vi "Untitled 1.vi"() -> ()   [LabVIEW 2019]
panel:
  out "Load Successful?":bool
  out "size(s)":i32
  in  "OK Button 2":bool
  out "element":string
  in  "Load new stations":bool
  in  "Line name":string
  in  "Line stations":string[](array[string])
  out "read buffer":string
  in  "VISA resource name":refnum<visa-resource-name>
  in  "Stop program":bool
  out "End\nStation":bool caption="N/A"
  out "Station 15":bool caption="N/A"
  out "Station 14":bool caption="N/A"
  out "Station 13":bool caption="N/A"
  out "Station 12":bool caption="N/A"
  out "Station 11":bool caption="N/A"
  out "Station 10":bool caption="N/A"
  out "Station 9":bool caption="N/A"
  out "Station 8":bool caption="N/A"
  out "Station 7":bool caption="sevsv"
  out "Station 6":bool caption="iugg"
  out "Station 5":bool caption="esceac"
  out "Station 4":bool caption="dwafa"
  out "Station 3":bool caption="wdca"
  out "Station 2":bool caption="kugiyg"
  out "Starting\nStation":bool caption="khfydug"
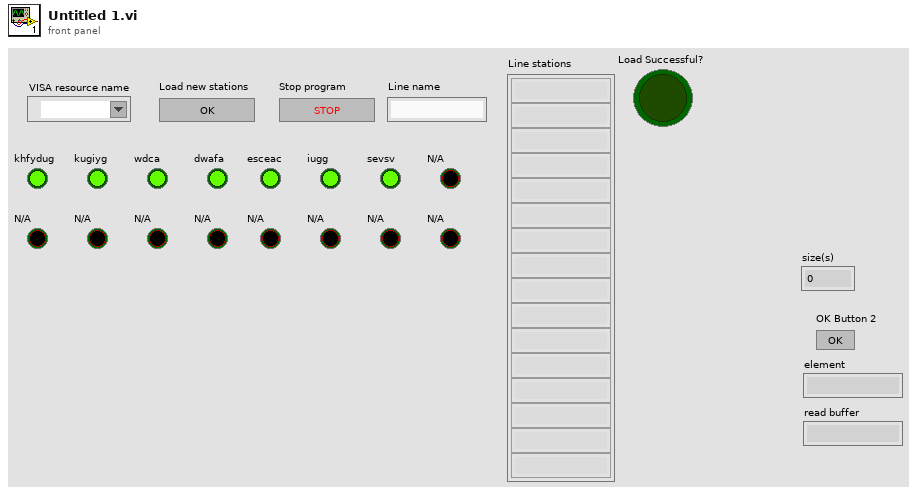
[diagram p1: front panel]
types:
  T1 = enum8{"Enabled", "Disabled", "Disabled and Grayed Out"}
  T2 = cluster{"[0]":bool, "[1]":bool, "[2]":bool, "[3]":bool, "[4]":bool, "[5]":bool, "[6]":bool, "[7]":bool, "[8]":bool}
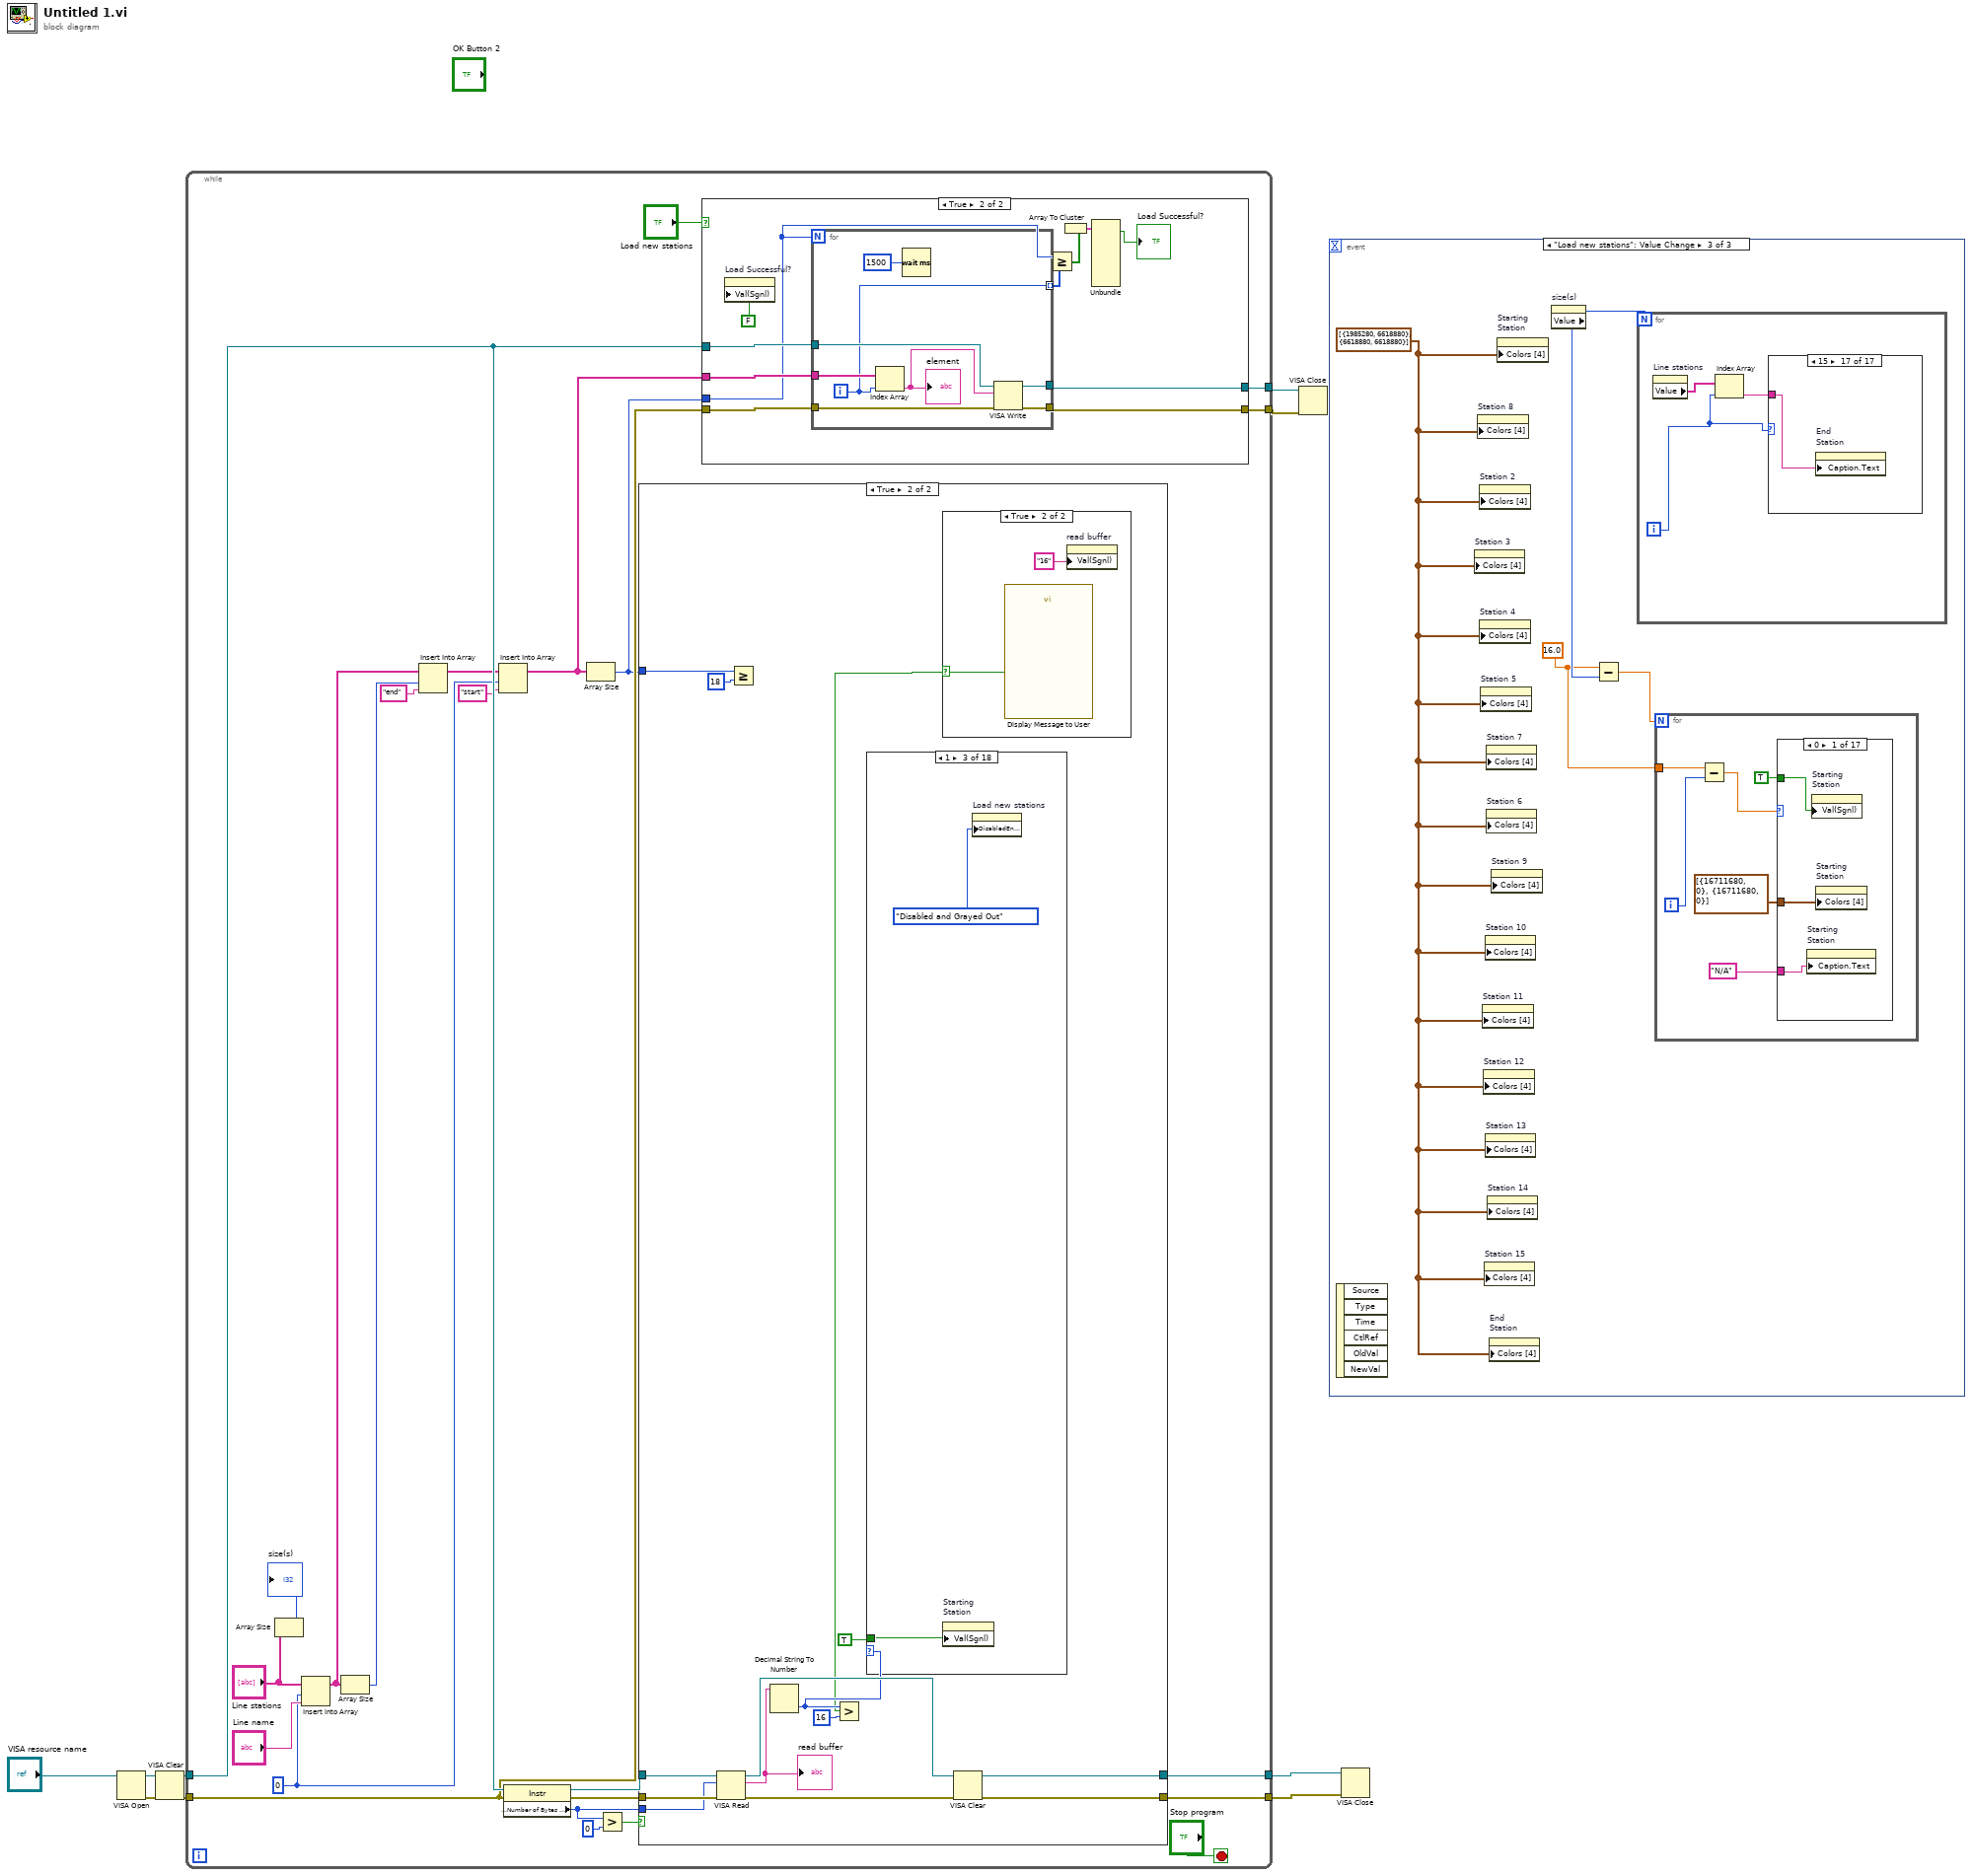
[diagram p0: block diagram]
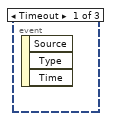
[diagram p2: hidden frame]
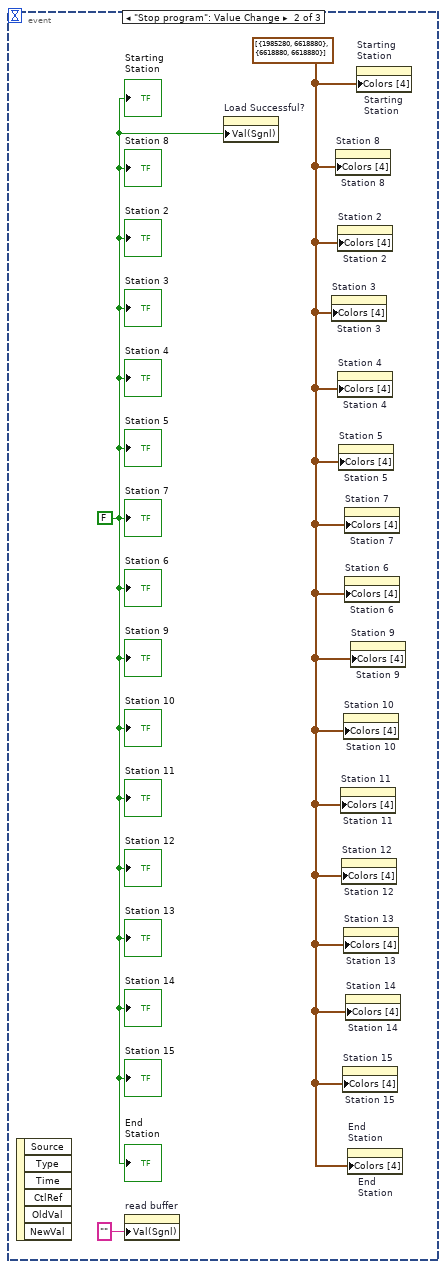
[diagram p3: hidden frame]
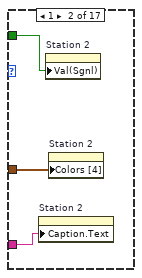
[diagram p4: hidden frame]
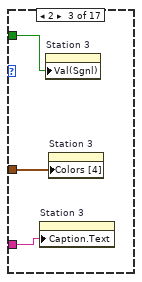
[diagram p5: hidden frame]
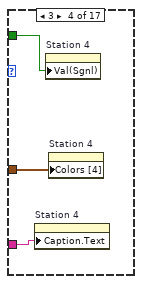
[diagram p6: hidden frame]
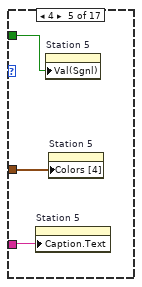
[diagram p7: hidden frame]
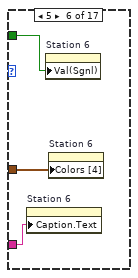
[diagram p8: hidden frame]
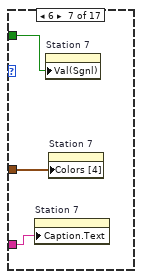
[diagram p9: hidden frame]
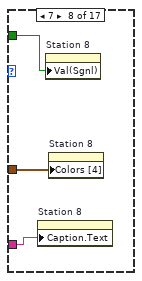
[diagram p10: hidden frame]
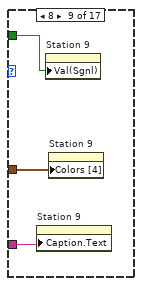
[diagram p11: hidden frame]
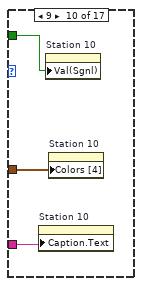
[diagram p12: hidden frame]
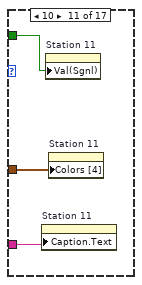
[diagram p13: hidden frame]
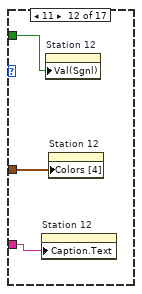
[diagram p14: hidden frame]
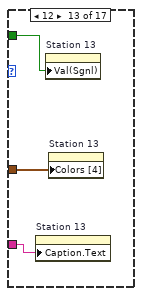
[diagram p15: hidden frame]
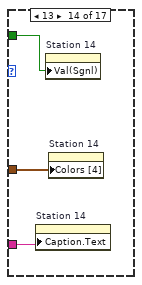
[diagram p16: hidden frame]
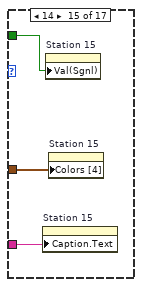
[diagram p17: hidden frame]
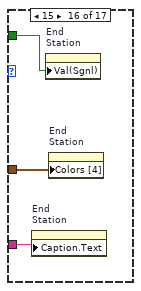
[diagram p18: hidden frame]
diagram:
  n1 = VISA Open(VISA resource name="VISA resource name") -> (VISA resource name=w5:refnum<visa-resource-name>, error out=w6:errorcluster)  [unwired: 4 in]
  n2 = VISA Clear(VISA resource name=w5, error in (no error)=w6) -> (VISA resource name out=w4:refnum<visa-resource-name>, error out=w3:errorcluster)
  n3 = while {
    tunnel: w4 -> [w21]
    tunnel: w3 -> [w20]
    tunnel: [w28] -> w8
    tunnel: [w27] -> w7
    tunnel: [w16] -> w2
    tunnel: [w15] -> w1
    stop <- "Stop program" stop-if-true
    w14 = 0 ("index")
    n4 = Array Size(array="Line stations") -> (size(s)=→"size(s)":i32)
    n5 = Insert Into Array(array="Line stations", index=w14, new element="Line name") -> (w22:string[])
    n6 = Array Size(array=w22) -> (size(s)=w23:i32)
    n7 = Insert Into Array(array=w22, index=w23, new element="end") -> (w18:string[])
    n8 = Insert Into Array(array=w18, index=w14, new element="start" ("new element/subarray")) -> (w13:string[])
    n9 = property class="Instr"(reference=w21, error in=w20) -> (reference out=w31:refnum<visa-resource-name>, error out=w30:errorcluster, "Serial Settings:Number of Bytes at Serial Port"=w29:u32)
    n10 = Array Size(array=w13) -> (size(s)=w12:i32)
    n11 = Greater?(x=w29, y=u32 0) -> (0:w32:bool)
    n12 = case shown="True" w32 {
      tunnel: w31 -> [w56 w70]
      tunnel: w30 -> [w55 w69]
      tunnel: [w56 w67] -> w27
      tunnel: [w55 w64] -> w28
      tunnel: w29 -> [_ w68]
      tunnel: w12 -> [_ w59]
      frame False {
      }
      frame True {
        n13 = VISA Read(VISA resource name=w70, byte count=w68, error in (no error)=w69) -> (VISA resource name out=w66:refnum<visa-resource-name>, read buffer=w63:string, error out=w65:errorcluster)  [unwired: 1 out]
        "read buffer" <- w63
        n14 = Greater Or Equal?(x=w59, y=18) -> ()  [unwired: 1 out]
        n15 = Decimal String To Number(string=w63) -> (number=w60:i32)  [unwired: 2 in, 1 out]
        n16 = Greater?(x=w60, y=16) -> (0:w57:bool)
        n17 = case shown="1" w60 {
          tunnel: TRUE -> [_ _ w76 w77 w78 w79 w80 w81 w82 w83 w84 w85 w86 w87 w88 w89 w90 w91]
          frame Default {
          }
          frame 0 {
            w73 = FALSE
            n18 = property on="Load new stations" class="Bool"("DisabledEnum"=T1."Enabled" ("Disabled")) -> ()  [unwired: 2 in, 2 out]
            n19 = property on="Station 5" class="Bool (strict)"("Val(Sgnl)"=w73) -> ()  [unwired: 2 in, 2 out]
            n20 = property on="Station 4" class="Bool (strict)"("Val(Sgnl)"=w73) -> ()  [unwired: 2 in, 2 out]
            n21 = property on="Station 6" class="Bool (strict)"("Val(Sgnl)"=w73) -> ()  [unwired: 2 in, 2 out]
            n22 = property on="Station 3" class="Bool (strict)"("Val(Sgnl)"=w73) -> ()  [unwired: 2 in, 2 out]
            n23 = property on="Starting\nStation" class="Bool (strict)"("Val(Sgnl)"=w73) -> ()  [unwired: 2 in, 2 out]
            n24 = property on="Station 2" class="Bool (strict)"("Val(Sgnl)"=w73) -> ()  [unwired: 2 in, 2 out]
            n25 = property on="Station 7" class="Bool (strict)"("Val(Sgnl)"=w73) -> ()  [unwired: 2 in, 2 out]
            n26 = property on="Station 11" class="Bool (strict)"("Val(Sgnl)"=w73) -> ()  [unwired: 2 in, 2 out]
            n27 = property on="Station 12" class="Bool (strict)"("Val(Sgnl)"=w73) -> ()  [unwired: 2 in, 2 out]
            n28 = property on="Station 10" class="Bool (strict)"("Val(Sgnl)"=w73) -> ()  [unwired: 2 in, 2 out]
            n29 = property on="Station 9" class="Bool (strict)"("Val(Sgnl)"=w73) -> ()  [unwired: 2 in, 2 out]
            n30 = property on="Station 8" class="Bool (strict)"("Val(Sgnl)"=w73) -> ()  [unwired: 2 in, 2 out]
            n31 = property on="Station 15" class="Bool (strict)"("Val(Sgnl)"=w73) -> ()  [unwired: 2 in, 2 out]
            n32 = property on="Station 13" class="Bool (strict)"("Val(Sgnl)"=w73) -> ()  [unwired: 2 in, 2 out]
            n33 = property on="End\nStation" class="Bool (strict)"("Val(Sgnl)"=w73) -> ()  [unwired: 2 in, 2 out]
            n34 = property on="Station 14" class="Bool (strict)"("Val(Sgnl)"=w73) -> ()  [unwired: 2 in, 2 out]
          }
          frame 1 {
            n35 = property on="Starting\nStation" class="Bool (strict)"("Val(Sgnl)"=w76) -> ()  [unwired: 2 in, 2 out]
            n36 = property on="Load new stations" class="Bool"("DisabledEnum"=T1."Disabled and Grayed Out" ("Disabled")) -> ()  [unwired: 2 in, 2 out]
          }
          frame 2 {
            n37 = property on="Station 2" class="Bool (strict)"("Val(Sgnl)"=w77) -> ()  [unwired: 2 in, 2 out]
          }
          frame 3 {
            n38 = property on="Station 3" class="Bool (strict)"("Val(Sgnl)"=w78) -> ()  [unwired: 2 in, 2 out]
          }
          frame 4 {
            n39 = property on="Station 4" class="Bool (strict)"("Val(Sgnl)"=w79) -> ()  [unwired: 2 in, 2 out]
          }
          frame 5 {
            n40 = property on="Station 5" class="Bool (strict)"("Val(Sgnl)"=w80) -> ()  [unwired: 2 in, 2 out]
          }
          frame 6 {
            n41 = property on="Station 6" class="Bool (strict)"("Val(Sgnl)"=w81) -> ()  [unwired: 2 in, 2 out]
          }
          frame 7 {
            n42 = property on="Station 7" class="Bool (strict)"("Val(Sgnl)"=w82) -> ()  [unwired: 2 in, 2 out]
          }
          frame 8 {
            n43 = property on="Station 8" class="Bool (strict)"("Val(Sgnl)"=w83) -> ()  [unwired: 2 in, 2 out]
          }
          frame 9 {
            n44 = property on="Station 9" class="Bool (strict)"("Val(Sgnl)"=w84) -> ()  [unwired: 2 in, 2 out]
          }
          frame 10 {
            n45 = property on="Station 10" class="Bool (strict)"("Val(Sgnl)"=w85) -> ()  [unwired: 2 in, 2 out]
          }
          frame 11 {
            n46 = property on="Station 11" class="Bool (strict)"("Val(Sgnl)"=w86) -> ()  [unwired: 2 in, 2 out]
          }
          frame 12 {
            n47 = property on="Station 12" class="Bool (strict)"("Val(Sgnl)"=w87) -> ()  [unwired: 2 in, 2 out]
          }
          frame 13 {
            n48 = property on="Station 13" class="Bool (strict)"("Val(Sgnl)"=w88) -> ()  [unwired: 2 in, 2 out]
          }
          frame 14 {
            n49 = property on="Station 14" class="Bool (strict)"("Val(Sgnl)"=w89) -> ()  [unwired: 2 in, 2 out]
          }
          frame 15 {
            n50 = property on="Station 15" class="Bool (strict)"("Val(Sgnl)"=w90) -> ()  [unwired: 2 in, 2 out]
          }
          frame 16 {
            n51 = property on="End\nStation" class="Bool (strict)"("Val(Sgnl)"=w91) -> ()  [unwired: 2 in, 2 out]
          }
        }
        n52 = case shown="True" w57 {
          selector: w57 -> [_ w72]
          frame False {
          }
          frame True {
            n53 = call "Display Message to User"("Enable"=w72) -> ()  [unwired: 9 in, 2 out]
            n54 = property on="read buffer" class="Str"("Val(Sgnl)"="16" ("Value (Signaling)")) -> ()  [unwired: 2 in, 2 out]
          }
        }
        n55 = VISA Clear(VISA resource name=w66, error in (no error)=w65) -> (VISA resource name out=w67:refnum<visa-resource-name>, error out=w64:errorcluster)
      }
    }
    n56 = case shown="True" "Load new stations" {
      tunnel: w21 -> [w35 w45]
      tunnel: w20 -> [w34 w44]
      tunnel: w13 -> [_ w46]
      tunnel: [w35 w43] -> w16
      tunnel: [w34 w42] -> w15
      tunnel: w12 -> [_ w41]
      frame False {
      }
      frame True {
        n57 = property on="Load Successful?" class="Bool (strict)"("Val(Sgnl)"=FALSE ("Value (Signaling)")) -> ()  [unwired: 2 in, 2 out]
        n58 = for {
          N: w41 -> [_]
          tunnel: w46 -> [w54]
          tunnel: w45 -> [w53]
          tunnel: w44 -> [w52]
          tunnel: [w50] -> w43
          tunnel: [w49] -> w42
          tunnel: [w47] -> w40 mode=indexing
          i -> [w47]
          n59 = Index Array(array=w54, index=w47) -> (element=w51:string)
          "element" <- w51
          n60 = Wait (ms)(milliseconds to wait=u32 1500) -> ()  [unwired: 1 out]
          n61 = VISA Write(VISA resource name=w53, write buffer=w51, error in (no error)=w52) -> (VISA resource name out=w50:refnum<visa-resource-name>, error out=w49:errorcluster)  [unwired: 1 out]
        }
        n62 = Greater Or Equal?(x=w41, y=w40) -> (x >= y?=w39:bool[])
        n63 = Array To Cluster(array=w39) -> (cluster=w38:T2)
        n64 = Unbundle(w38) -> ("[1]"=→"Load Successful?":bool)  [unwired: 8 out]
      }
    }
  }
  n65 = VISA Close(VISA resource name=w2, error in (no error)=w1) -> ()  [unwired: 1 out]
  n66 = event shown="[2] \"Load new stations\": Value Change" {
    selector: _ -> [_ _ _]
    dyn-events: _ -> [_ _ _]
    timeout: _ -> [_ _ _]
    event Timeout {
      n67 = event-data() -> ()  [unwired: 1 in, 3 out]
    }
    event "Stop program": Value Change {
      w93 = cluster{u32, u32}[] [{1985280, 6618880}, {6618880, 6618880}] ("Colors [4]")
      w94 = cluster{u32, u32}[] [{1985280, 6618880}, {6618880, 6618880}] ("Colors [4]")
      w92 = FALSE
      n68 = event-data() -> ()  [unwired: 1 in, 6 out]
      n69 = property on="read buffer" class="Str"("Val(Sgnl)"="" ("Value (Signaling)")) -> ()  [unwired: 2 in, 2 out]
      n70 = property on="Load Successful?" class="Bool (strict)"("Val(Sgnl)"=w92) -> ()  [unwired: 2 in, 2 out]
      n71 = property on="Station 3" class="Bool (strict)"("Colors [4]"=w93) -> ()  [unwired: 2 in, 2 out]
      n72 = property on="Station 3" class="Bool (strict)"("Colors [4]"=w94) -> ()  [unwired: 2 in, 2 out]
      n73 = property on="Station 8" class="Bool (strict)"("Colors [4]"=w93) -> ()  [unwired: 2 in, 2 out]
      n74 = property on="Station 8" class="Bool (strict)"("Colors [4]"=w94) -> ()  [unwired: 2 in, 2 out]
      n75 = property on="Station 2" class="Bool (strict)"("Colors [4]"=w93) -> ()  [unwired: 2 in, 2 out]
      n76 = property on="Station 2" class="Bool (strict)"("Colors [4]"=w94) -> ()  [unwired: 2 in, 2 out]
      n77 = property on="Station 4" class="Bool (strict)"("Colors [4]"=w93) -> ()  [unwired: 2 in, 2 out]
      n78 = property on="Station 4" class="Bool (strict)"("Colors [4]"=w94) -> ()  [unwired: 2 in, 2 out]
      n79 = property on="Station 5" class="Bool (strict)"("Colors [4]"=w93) -> ()  [unwired: 2 in, 2 out]
      n80 = property on="Station 5" class="Bool (strict)"("Colors [4]"=w94) -> ()  [unwired: 2 in, 2 out]
      n81 = property on="Station 11" class="Bool (strict)"("Colors [4]"=w93) -> ()  [unwired: 2 in, 2 out]
      n82 = property on="Station 11" class="Bool (strict)"("Colors [4]"=w94) -> ()  [unwired: 2 in, 2 out]
      n83 = property on="Station 12" class="Bool (strict)"("Colors [4]"=w93) -> ()  [unwired: 2 in, 2 out]
      n84 = property on="Station 12" class="Bool (strict)"("Colors [4]"=w94) -> ()  [unwired: 2 in, 2 out]
      n85 = property on="Station 15" class="Bool (strict)"("Colors [4]"=w93) -> ()  [unwired: 2 in, 2 out]
      n86 = property on="Station 15" class="Bool (strict)"("Colors [4]"=w94) -> ()  [unwired: 2 in, 2 out]
      n87 = property on="Station 10" class="Bool (strict)"("Colors [4]"=w93) -> ()  [unwired: 2 in, 2 out]
      n88 = property on="Station 10" class="Bool (strict)"("Colors [4]"=w94) -> ()  [unwired: 2 in, 2 out]
      n89 = property on="Station 13" class="Bool (strict)"("Colors [4]"=w93) -> ()  [unwired: 2 in, 2 out]
      n90 = property on="Station 13" class="Bool (strict)"("Colors [4]"=w94) -> ()  [unwired: 2 in, 2 out]
      n91 = property on="Station 7" class="Bool (strict)"("Colors [4]"=w93) -> ()  [unwired: 2 in, 2 out]
      n92 = property on="Station 7" class="Bool (strict)"("Colors [4]"=w94) -> ()  [unwired: 2 in, 2 out]
      n93 = property on="Station 6" class="Bool (strict)"("Colors [4]"=w93) -> ()  [unwired: 2 in, 2 out]
      n94 = property on="Station 6" class="Bool (strict)"("Colors [4]"=w94) -> ()  [unwired: 2 in, 2 out]
      n95 = property on="Station 14" class="Bool (strict)"("Colors [4]"=w93) -> ()  [unwired: 2 in, 2 out]
      n96 = property on="Station 14" class="Bool (strict)"("Colors [4]"=w94) -> ()  [unwired: 2 in, 2 out]
      n97 = property on="End\nStation" class="Bool (strict)"("Colors [4]"=w93) -> ()  [unwired: 2 in, 2 out]
      n98 = property on="End\nStation" class="Bool (strict)"("Colors [4]"=w94) -> ()  [unwired: 2 in, 2 out]
      n99 = property on="Station 9" class="Bool (strict)"("Colors [4]"=w93) -> ()  [unwired: 2 in, 2 out]
      n100 = property on="Station 9" class="Bool (strict)"("Colors [4]"=w94) -> ()  [unwired: 2 in, 2 out]
      n101 = property on="Starting\nStation" class="Bool (strict)"("Colors [4]"=w93) -> ()  [unwired: 2 in, 2 out]
      n102 = property on="Starting\nStation" class="Bool (strict)"("Colors [4]"=w94) -> ()  [unwired: 2 in, 2 out]
      "Station 2" <- w92
      "Station 3" <- w92
      "Station 4" <- w92
      "Station 5" <- w92
      "Station 6" <- w92
      "Station 7" <- w92
      "Station 8" <- w92
      "Station 9" <- w92
      "Station 10" <- w92
      "Station 11" <- w92
      "Station 12" <- w92
      "Station 13" <- w92
      "Station 14" <- w92
      "Station 15" <- w92
      "End\nStation" <- w92
      "Starting\nStation" <- w92
    }
    event "Load new stations": Value Change {
      w96 = cluster{u32, u32}[] [{1985280, 6618880}, {6618880, 6618880}] ("Colors [4]")
      w97 = 16.0 ("x")
      n103 = event-data() -> ()  [unwired: 1 in, 6 out]
      n104 = property on="Station 3" class="Bool (strict)"("Colors [4]"=w96) -> ()  [unwired: 2 in, 2 out]
      n105 = property on="Station 8" class="Bool (strict)"("Colors [4]"=w96) -> ()  [unwired: 2 in, 2 out]
      n106 = property on="Station 2" class="Bool (strict)"("Colors [4]"=w96) -> ()  [unwired: 2 in, 2 out]
      n107 = property on="Station 4" class="Bool (strict)"("Colors [4]"=w96) -> ()  [unwired: 2 in, 2 out]
      n108 = property on="Station 5" class="Bool (strict)"("Colors [4]"=w96) -> ()  [unwired: 2 in, 2 out]
      n109 = property on="Station 11" class="Bool (strict)"("Colors [4]"=w96) -> ()  [unwired: 2 in, 2 out]
      n110 = property on="Station 12" class="Bool (strict)"("Colors [4]"=w96) -> ()  [unwired: 2 in, 2 out]
      n111 = property on="Station 15" class="Bool (strict)"("Colors [4]"=w96) -> ()  [unwired: 2 in, 2 out]
      n112 = property on="Station 10" class="Bool (strict)"("Colors [4]"=w96) -> ()  [unwired: 2 in, 2 out]
      n113 = property on="Station 13" class="Bool (strict)"("Colors [4]"=w96) -> ()  [unwired: 2 in, 2 out]
      n114 = property on="Station 7" class="Bool (strict)"("Colors [4]"=w96) -> ()  [unwired: 2 in, 2 out]
      n115 = property on="Station 6" class="Bool (strict)"("Colors [4]"=w96) -> ()  [unwired: 2 in, 2 out]
      n116 = property on="Station 14" class="Bool (strict)"("Colors [4]"=w96) -> ()  [unwired: 2 in, 2 out]
      n117 = property on="End\nStation" class="Bool (strict)"("Colors [4]"=w96) -> ()  [unwired: 2 in, 2 out]
      n118 = property on="Station 9" class="Bool (strict)"("Colors [4]"=w96) -> ()  [unwired: 2 in, 2 out]
      n119 = property on="Starting\nStation" class="Bool (strict)"("Colors [4]"=w96) -> ()  [unwired: 2 in, 2 out]
      n120 = property on="size(s)" class="DigNum (strict)"() -> ("Value"=w99:i32)  [unwired: 2 in, 2 out]
      n121 = Subtract(x=w97, y=w99) -> (x-y=w98:dbl)
      n122 = for {
        N: w99 -> [_]
        i -> [w154]
        n123 = property on="Line stations" class="Arr (strict)"() -> ("Value"=w156:string[])  [unwired: 2 in, 2 out]
        n124 = Index Array(array=w156, index=w154) -> (element=w155:string)
        n125 = case shown="15" w154 {
          tunnel: w155 -> [_ w157 w158 w159 w160 w161 w162 w163 w164 w165 w166 w167 w168 w169 w170 w171 w172]
          frame Default {
          }
          frame 0 {
            n126 = property on="Starting\nStation" class="Bool (strict)"("Caption.Text"=w157) -> ()  [unwired: 2 in, 2 out]
          }
          frame 1 {
            n127 = property on="Station 2" class="Bool (strict)"("Caption.Text"=w158) -> ()  [unwired: 2 in, 2 out]
          }
          frame 2 {
            n128 = property on="Station 3" class="Bool (strict)"("Caption.Text"=w159) -> ()  [unwired: 2 in, 2 out]
          }
          frame 3 {
            n129 = property on="Station 4" class="Bool (strict)"("Caption.Text"=w160) -> ()  [unwired: 2 in, 2 out]
          }
          frame 4 {
            n130 = property on="Station 5" class="Bool (strict)"("Caption.Text"=w161) -> ()  [unwired: 2 in, 2 out]
          }
          frame 5 {
            n131 = property on="Station 6" class="Bool (strict)"("Caption.Text"=w162) -> ()  [unwired: 2 in, 2 out]
          }
          frame 6 {
            n132 = property on="Station 7" class="Bool (strict)"("Caption.Text"=w163) -> ()  [unwired: 2 in, 2 out]
          }
          frame 7 {
            n133 = property on="Station 8" class="Bool (strict)"("Caption.Text"=w164) -> ()  [unwired: 2 in, 2 out]
          }
          frame 8 {
            n134 = property on="Station 9" class="Bool (strict)"("Caption.Text"=w165) -> ()  [unwired: 2 in, 2 out]
          }
          frame 9 {
            n135 = property on="Station 10" class="Bool (strict)"("Caption.Text"=w166) -> ()  [unwired: 2 in, 2 out]
          }
          frame 10 {
            n136 = property on="Station 11" class="Bool (strict)"("Caption.Text"=w167) -> ()  [unwired: 2 in, 2 out]
          }
          frame 11 {
            n137 = property on="Station 12" class="Bool (strict)"("Caption.Text"=w168) -> ()  [unwired: 2 in, 2 out]
          }
          frame 12 {
            n138 = property on="Station 13" class="Bool (strict)"("Caption.Text"=w169) -> ()  [unwired: 2 in, 2 out]
          }
          frame 13 {
            n139 = property on="Station 14" class="Bool (strict)"("Caption.Text"=w170) -> ()  [unwired: 2 in, 2 out]
          }
          frame 14 {
            n140 = property on="Station 15" class="Bool (strict)"("Caption.Text"=w171) -> ()  [unwired: 2 in, 2 out]
          }
          frame 15 {
            n141 = property on="End\nStation" class="Bool (strict)"("Caption.Text"=w172) -> ()  [unwired: 2 in, 2 out]
          }
        }
      }
      n142 = for {
        N: w98 -> [_]
        tunnel: w97 -> [w105]
        i -> [w104]
        n143 = Subtract(x=w105, y=w104) -> (x-y=w103:dbl)
        n144 = case shown="0" w103 {
          tunnel: cluster{u32, u32}[] [{16711680, 0}, {16711680, 0}] ("Colors [4]") -> [w108 w111 w114 w117 w120 w123 w126 w129 w132 w135 w138 w141 w144 w147 w150 w153 _]
          tunnel: TRUE ("Value (Signaling)") -> [w107 w110 w113 w116 w119 w122 w125 w128 w131 w134 w137 w140 w143 w146 w149 w152 _]
          tunnel: "N/A" ("Caption.Text") -> [w106 w109 w112 w115 w118 w121 w124 w127 w130 w133 w136 w139 w142 w145 w148 w151 _]
          frame 0 {
            n145 = property on="Starting\nStation" class="Bool (strict)"("Caption.Text"=w106) -> ()  [unwired: 2 in, 2 out]
            n146 = property on="Starting\nStation" class="Bool (strict)"("Val(Sgnl)"=w107) -> ()  [unwired: 2 in, 2 out]
            n147 = property on="Starting\nStation" class="Bool (strict)"("Colors [4]"=w108) -> ()  [unwired: 2 in, 2 out]
          }
          frame 1 {
            n148 = property on="Station 2" class="Bool (strict)"("Caption.Text"=w109) -> ()  [unwired: 2 in, 2 out]
            n149 = property on="Station 2" class="Bool (strict)"("Val(Sgnl)"=w110) -> ()  [unwired: 2 in, 2 out]
            n150 = property on="Station 2" class="Bool (strict)"("Colors [4]"=w111) -> ()  [unwired: 2 in, 2 out]
          }
          frame 2 {
            n151 = property on="Station 3" class="Bool (strict)"("Caption.Text"=w112) -> ()  [unwired: 2 in, 2 out]
            n152 = property on="Station 3" class="Bool (strict)"("Val(Sgnl)"=w113) -> ()  [unwired: 2 in, 2 out]
            n153 = property on="Station 3" class="Bool (strict)"("Colors [4]"=w114) -> ()  [unwired: 2 in, 2 out]
          }
          frame 3 {
            n154 = property on="Station 4" class="Bool (strict)"("Caption.Text"=w115) -> ()  [unwired: 2 in, 2 out]
            n155 = property on="Station 4" class="Bool (strict)"("Val(Sgnl)"=w116) -> ()  [unwired: 2 in, 2 out]
            n156 = property on="Station 4" class="Bool (strict)"("Colors [4]"=w117) -> ()  [unwired: 2 in, 2 out]
          }
          frame 4 {
            n157 = property on="Station 5" class="Bool (strict)"("Caption.Text"=w118) -> ()  [unwired: 2 in, 2 out]
            n158 = property on="Station 5" class="Bool (strict)"("Val(Sgnl)"=w119) -> ()  [unwired: 2 in, 2 out]
            n159 = property on="Station 5" class="Bool (strict)"("Colors [4]"=w120) -> ()  [unwired: 2 in, 2 out]
          }
          frame 5 {
            n160 = property on="Station 6" class="Bool (strict)"("Caption.Text"=w121) -> ()  [unwired: 2 in, 2 out]
            n161 = property on="Station 6" class="Bool (strict)"("Val(Sgnl)"=w122) -> ()  [unwired: 2 in, 2 out]
            n162 = property on="Station 6" class="Bool (strict)"("Colors [4]"=w123) -> ()  [unwired: 2 in, 2 out]
          }
          frame 6 {
            n163 = property on="Station 7" class="Bool (strict)"("Caption.Text"=w124) -> ()  [unwired: 2 in, 2 out]
            n164 = property on="Station 7" class="Bool (strict)"("Val(Sgnl)"=w125) -> ()  [unwired: 2 in, 2 out]
            n165 = property on="Station 7" class="Bool (strict)"("Colors [4]"=w126) -> ()  [unwired: 2 in, 2 out]
          }
          frame 7 {
            n166 = property on="Station 8" class="Bool (strict)"("Caption.Text"=w127) -> ()  [unwired: 2 in, 2 out]
            n167 = property on="Station 8" class="Bool (strict)"("Val(Sgnl)"=w128) -> ()  [unwired: 2 in, 2 out]
            n168 = property on="Station 8" class="Bool (strict)"("Colors [4]"=w129) -> ()  [unwired: 2 in, 2 out]
          }
          frame 8 {
            n169 = property on="Station 9" class="Bool (strict)"("Caption.Text"=w130) -> ()  [unwired: 2 in, 2 out]
            n170 = property on="Station 9" class="Bool (strict)"("Val(Sgnl)"=w131) -> ()  [unwired: 2 in, 2 out]
            n171 = property on="Station 9" class="Bool (strict)"("Colors [4]"=w132) -> ()  [unwired: 2 in, 2 out]
          }
          frame 9 {
            n172 = property on="Station 10" class="Bool (strict)"("Caption.Text"=w133) -> ()  [unwired: 2 in, 2 out]
            n173 = property on="Station 10" class="Bool (strict)"("Val(Sgnl)"=w134) -> ()  [unwired: 2 in, 2 out]
            n174 = property on="Station 10" class="Bool (strict)"("Colors [4]"=w135) -> ()  [unwired: 2 in, 2 out]
          }
          frame 10 {
            n175 = property on="Station 11" class="Bool (strict)"("Caption.Text"=w136) -> ()  [unwired: 2 in, 2 out]
            n176 = property on="Station 11" class="Bool (strict)"("Val(Sgnl)"=w137) -> ()  [unwired: 2 in, 2 out]
            n177 = property on="Station 11" class="Bool (strict)"("Colors [4]"=w138) -> ()  [unwired: 2 in, 2 out]
          }
          frame 11 {
            n178 = property on="Station 12" class="Bool (strict)"("Caption.Text"=w139) -> ()  [unwired: 2 in, 2 out]
            n179 = property on="Station 12" class="Bool (strict)"("Val(Sgnl)"=w140) -> ()  [unwired: 2 in, 2 out]
            n180 = property on="Station 12" class="Bool (strict)"("Colors [4]"=w141) -> ()  [unwired: 2 in, 2 out]
          }
          frame 12 {
            n181 = property on="Station 13" class="Bool (strict)"("Caption.Text"=w142) -> ()  [unwired: 2 in, 2 out]
            n182 = property on="Station 13" class="Bool (strict)"("Val(Sgnl)"=w143) -> ()  [unwired: 2 in, 2 out]
            n183 = property on="Station 13" class="Bool (strict)"("Colors [4]"=w144) -> ()  [unwired: 2 in, 2 out]
          }
          frame 13 {
            n184 = property on="Station 14" class="Bool (strict)"("Caption.Text"=w145) -> ()  [unwired: 2 in, 2 out]
            n185 = property on="Station 14" class="Bool (strict)"("Val(Sgnl)"=w146) -> ()  [unwired: 2 in, 2 out]
            n186 = property on="Station 14" class="Bool (strict)"("Colors [4]"=w147) -> ()  [unwired: 2 in, 2 out]
          }
          frame 14 {
            n187 = property on="Station 15" class="Bool (strict)"("Caption.Text"=w148) -> ()  [unwired: 2 in, 2 out]
            n188 = property on="Station 15" class="Bool (strict)"("Val(Sgnl)"=w149) -> ()  [unwired: 2 in, 2 out]
            n189 = property on="Station 15" class="Bool (strict)"("Colors [4]"=w150) -> ()  [unwired: 2 in, 2 out]
          }
          frame 15 {
            n190 = property on="End\nStation" class="Bool (strict)"("Caption.Text"=w151) -> ()  [unwired: 2 in, 2 out]
            n191 = property on="End\nStation" class="Bool (strict)"("Val(Sgnl)"=w152) -> ()  [unwired: 2 in, 2 out]
            n192 = property on="End\nStation" class="Bool (strict)"("Colors [4]"=w153) -> ()  [unwired: 2 in, 2 out]
          }
          frame 16, Default {
          }
        }
      }
    }
  }
  n193 = VISA Close(VISA resource name=w7, error in (no error)=w8) -> ()  [unwired: 1 out]
